vi "Init.vi"(8 "error in":errorcluster, 11 "MCU in":refnum<class "HSU MCU V2 Monitor CFG.lvclass">) -> (0 "error out":errorcluster, 3 "MCU out":refnum<class "HSU MCU V2 Monitor CFG.lvclass">)   [LabVIEW 2023, in "HSU MCU V2 Monitor CFG.lvclass"]
uses:
  HSU MCU V2 Monitor CFG.lvclass
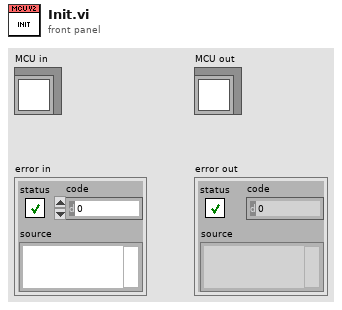
[diagram p1: front panel]
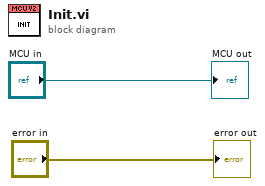
[diagram p0: block diagram]
diagram:
  "error out" <- "error in"
  "MCU out" <- "MCU in"
